vi "Set Top Level.vi"(6 "Variant in":variant, 7 "Shift Pressed?":bool, 8 "error in (no error)":errorcluster, 10 "QD Combo Box Ref":refnum<vi>, 11 "QD Launch VI Ref":refnum<vi>) -> (0 "error out":errorcluster, 4 "Variant out":variant)   [LabVIEW 2020]
doc: "Mark a VI in the project as the top level VI TopVI.\n\nDefault Shortcut - [M]"
panel:
  in  "Undo Name":string="Quick Drop Keyboard Shortcut"
  # "Do not change the connector pane of this VI.\n\nSee the block diagram for directions on how to use this template."
  # "Specify the name of the Undo transaction"
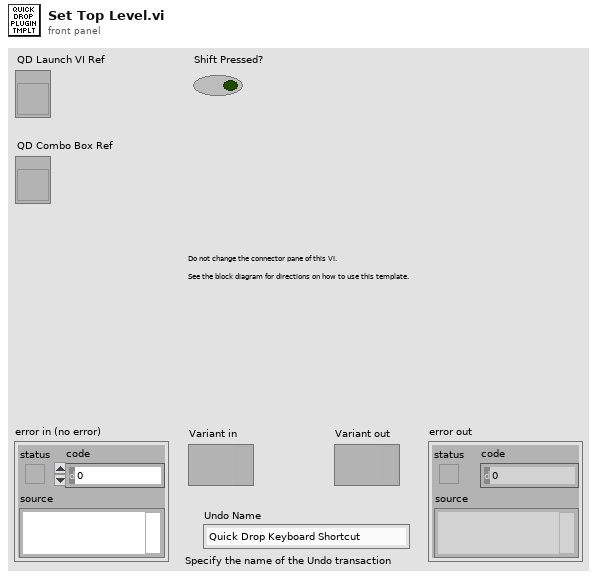
[diagram p1: front panel]
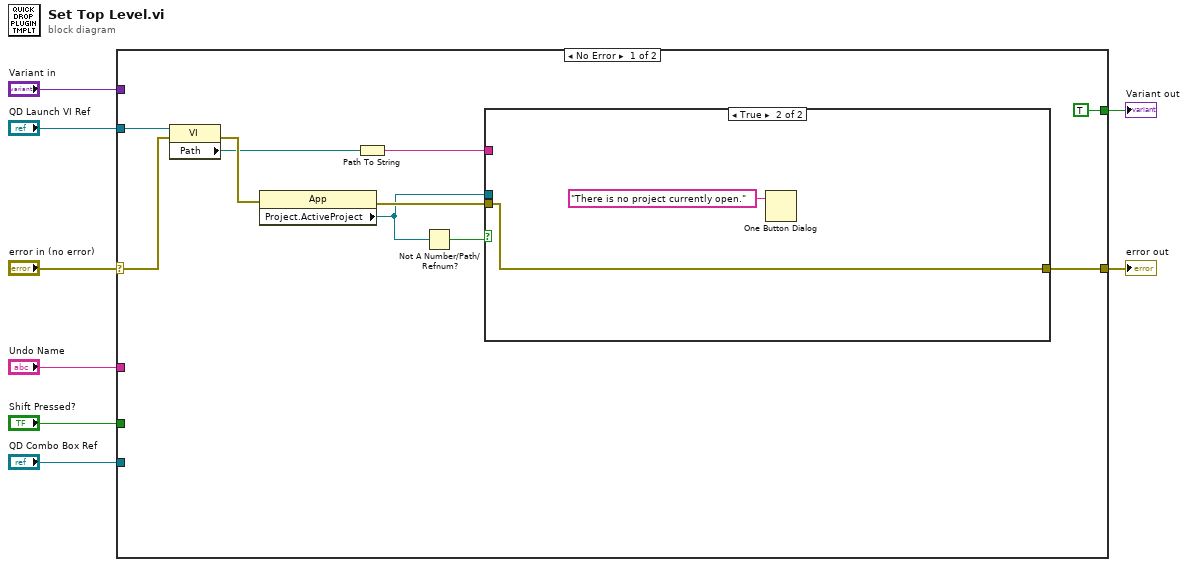
[diagram p0: block diagram]
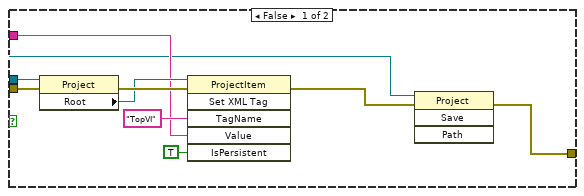
[diagram p2: hidden frame]
diagram:
  n1 = case shown="No Error" "error in (no error)" {
    selector: "error in (no error)" -> [w15 w30]
    tunnel: [w11 w30] -> w7
    tunnel: "QD Launch VI Ref" -> [w16 _]
    tunnel: "Shift Pressed?" -> [_ _]
    tunnel: "QD Combo Box Ref" -> [_ _]
    tunnel: "Variant in" -> [_ _]
    tunnel: "Undo Name" -> [_ _]
    tunnel: [TRUE _] -> w1
    frame No Error {
      n2 = property class="VI"(reference=w16, error in=w15) -> (error out=w14:errorcluster, "Path"=w13:path)  [unwired: 1 out]
      n3 = property class="App"(error in=w14) -> (error out=w17:errorcluster, "Project.ActiveProject"=w10:refnum<vi>)  [unwired: 1 in, 1 out]
      n4 = Path To String(path=w13) -> (string=w12:string)
      n5 = Not A Number/Path/Refnum?(number/path/refnum=w10) -> (NaN/Path/Refnum?=w9:bool)
      n6 = case shown="True" w9 {
        tunnel: w17 -> [w27 w28]
        tunnel: w12 -> [w22 _]
        tunnel: [w20 w28] -> w11
        tunnel: w10 -> [w19 _]
        frame False {
          n7 = property class="Project"(reference=w19, error in=w27) -> (error out=w26:errorcluster, "Root"=w25:refnum<vi>)  [unwired: 1 out]
          n8 = invoke class="ProjectItem" method="Set XML Tag"(reference=w25, error in=w26, "TagName"="TopVI" ("Tag Name"), "Value"=w22, "IsPersistent"=TRUE ("Is Persistent")) -> (error out=w21:errorcluster)  [unwired: 1 in, 5 out]
          n9 = invoke class="Project" method="Save"(reference=w19, error in=w21) -> (error out=w20:errorcluster)  [unwired: 2 in, 3 out]
        }
        frame True {
          n10 = One Button Dialog(message="There is no project currently open.") -> ()  [unwired: 1 in, 1 out]
        }
      }
    }
    frame Error {
    }
  }
  "error out" <- w7
  "Variant out" <- w1
